vi "GetInputTypeString.vi"(8 "error in (no error)":errorcluster, 10 "index":i32, 11 "session id in":i32) -> (0 "error out":errorcluster, 1 "InputTypeName":string, 2 "GetInputType":bool, 3 "session id out":i32)   [LabVIEW 2017, in "libonnx_wrapper.lvlib"]
doc: "/**\n * @brief Получить имя типа данных входа в виде строки\n * \n * Возвращает человекочитаемое имя типа данных (например, \"FLOAT32\", \"INT64\").\n * Удобно для отображения в интерфейсе LabVIEW и логирования.\n * \n * @param sessionId [IN] ID сессии\n * @param inputIndex [IN] Индекс входа (0-based)\n * @param buffer [OUT] Буфер для строки с именем типа\n * @param bufferSize [IN] Размер буфера в байтах (рекомендуется 32 или больше)\n * \n * @return int32: 0 при успешном копировании имени типа\n * @return int32: -1 если сессия не найдена или индекс неверен\n * \n * @note Возможные значения: \"FLOAT32\", \"FLOAT64\", \"INT8\", \"INT16\", \"INT32\", \n * \"INT64\", \"UINT8\", \"UINT16\", \"UINT32\", \"UINT64\", \"FLOAT16\", \"UNKNOWN\"\n */\nint GetInputTypeString(int sessionId, int inputIndex, char* buffer, int bufferSize);"
uses:
  libonnx_wrapper.lvlib
panel:
  out "bufferSize":i32
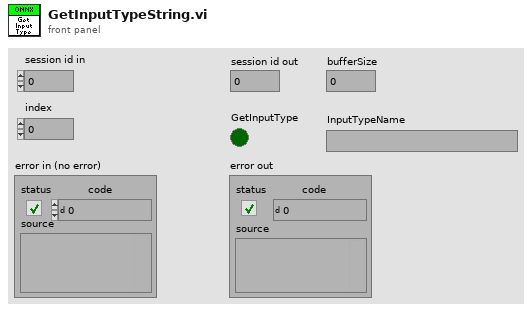
[diagram p1: front panel]
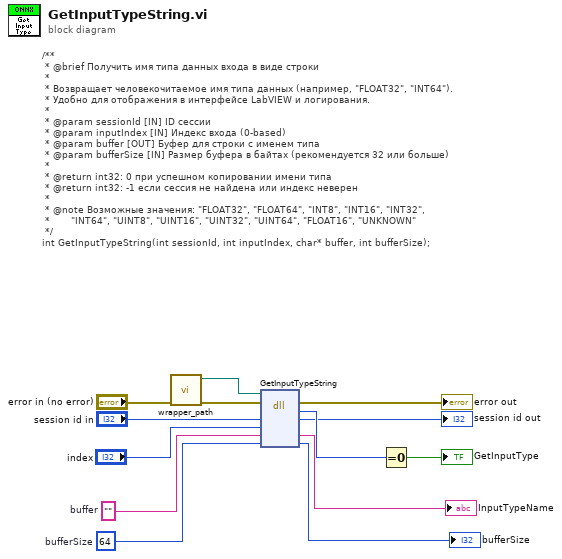
[diagram p0: block diagram]
diagram:
  w9 = 64  # bufferSize
  w11 = ""  # buffer
  # "/**\n * @brief Получить имя типа данных входа в виде строки\n * \n * Возвращает человекочитаемое имя типа данных (например, \"FLOAT32\", \"INT64\").\n * Удобно для отображения в интерфейсе LabVIEW и логирования.\n * \n * @param sessionId [IN] ID сессии\n * @param inputIndex [IN] Индекс входа (0-based)\n * @param buffer [OUT] Буфер для строки с именем типа\n * @param bufferSize [IN] Размер буфера в байтах (рекомендуется 32 или больше)\n * \n * @return int32: 0 при успешном копировании имени типа\n * @return int32: -1 если сессия не найдена или индекс неверен\n * \n * @note Возможные значения: \"FLOAT32\", \"FLOAT64\", \"INT8\", \"INT16\", \"INT32\", \n *       \"INT64\", \"UINT8\", \"UINT16\", \"UINT32\", \"UINT64\", \"FLOAT16\", \"UNKNOWN\"\n */\nint GetInputTypeString(int sessionId, int inputIndex, char* buffer, int bufferSize);"
  n1 = call "wrapper_path.vi"("error in (no error)"="error in (no error)") -> ("error out"=w4:errorcluster, "wrapper path"=w7:path)  [unwired: 9 in]
  n2 = dll-call lib="home/ivan/LabVIEWData/ONNX/Test/libonnx_wrapper/unix64/libonnx_wrapper.so" fn="GetInputTypeString"(path in=w7, error in=w4, "sessionId"="session id in", "inputIndex"="index", "buffer"=w11, "bufferSize"=w9) -> (error out=→"error out":errorcluster, "GetInputType"=w13:i32, "sessionId"=→"session id out":i32, "buffer"=→"InputTypeName":string, "bufferSize"=→"bufferSize":i32)  [unwired: 2 in, 1 out]
  n3 = Equal To 0?(x=w13) -> (x = 0?=→"GetInputType":bool)
